vi "Write bangBangParameters.vi"(8 "error in (no error)":errorcluster, 10 "bangBangParameters":T1={"MaxVSent"=6.5, "MaxVNorm"=1.0, "MaxVAng"=3.0, "VAngCircle"=2.5, "LBeginCircle"=300.0, "DistToDestOrientation"=400.0, "MaxVAngToTurn"=5.0, "AtkDistToDestOrientation"=4000.0, "KepperMaxVSent"=6.5, "VelNearEnemy"=1.5}, 11 "Parameters in":refnum<class "Parameters.lvclass">) -> (0 "error out":errorcluster, 3 "Parameters out":refnum<class "Parameters.lvclass">)   [LabVIEW 2023, in "Parameters.lvclass"]
uses:
  Parameters.lvclass
  Game_class/Navigation/Controls/bangBangControlParameters.ctl
  Parameters.lvclass/Parameters.ctl
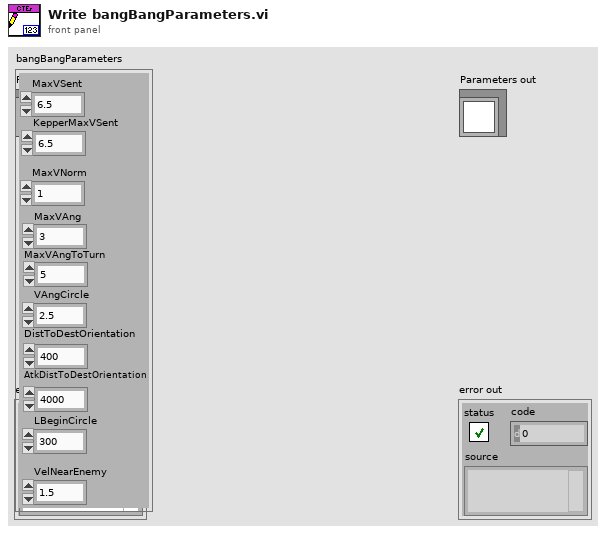
[diagram p1: front panel]
types:
  T1 = typedef "bangBangControlParameters.ctl" = cluster{"MaxVSent":dbl, "MaxVNorm":dbl, "MaxVAng":dbl, "VAngCircle":dbl, "LBeginCircle":dbl, "DistToDestOrientation":dbl, "MaxVAngToTurn":dbl, "AtkDistToDestOrientation":dbl, "KepperMaxVSent":dbl, "VelNearEnemy":dbl}
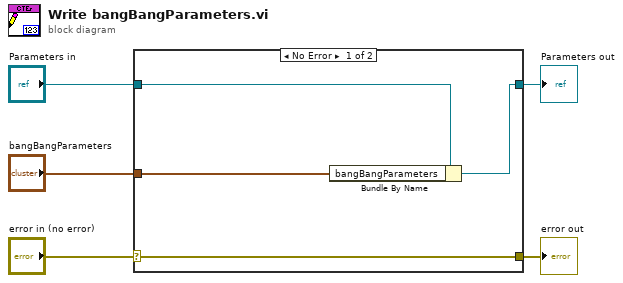
[diagram p0: block diagram]
diagram:
  n1 = case shown="No Error" "error in (no error)" {
    selector: "error in (no error)" -> [w9 w10]
    tunnel: [w9 w10] -> w4
    tunnel: [w7 w11] -> w2
    tunnel: "Parameters in" -> [w8 w11]
    tunnel: "bangBangParameters" -> [w6 _]
    frame No Error {
      n2 = Bundle By Name(cluster=w8, "bangBangParameters"=w6) -> (w7:refnum<class "Parameters.lvclass">)
    }
    frame Error {
    }
  }
  "error out" <- w4
  "Parameters out" <- w2
